vi "sort_according_to_x.vi"(8 "error in (no error)":errorcluster, 10 "points in":refnum<class "SpaceVector.lvclass">[](array[class])) -> (0 "error out":errorcluster, 2 "points out":refnum<class "SpaceVector.lvclass">[](array[class]))   [LabVIEW 2010, in "TrajectoryDL121017Hopping.lvclass"]
doc: "Sorts points according to their x coordinate."
uses:
  TrajectoryDL121017Hopping.lvclass
  common/classes/SpaceVector/SpaceVector/SpaceVector.lvclass
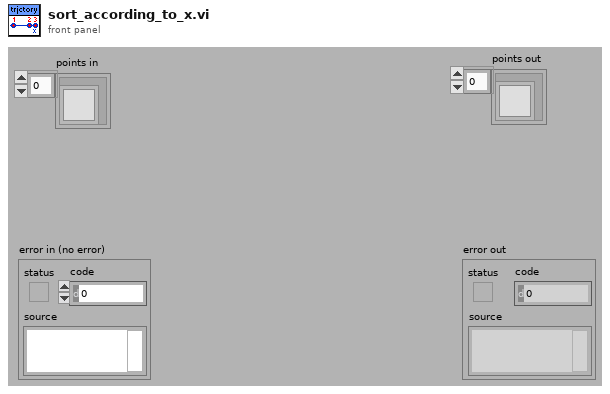
[diagram p1: front panel]
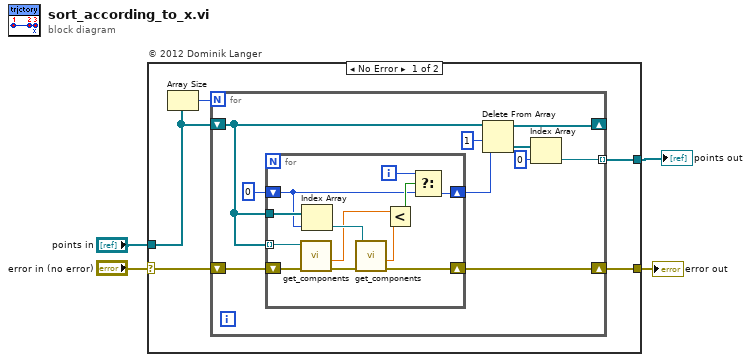
[diagram p0: block diagram]
diagram:
  n1 = case "© 2012 Dominik Langer" shown="No Error" "error in (no error)" {
    selector: "error in (no error)" -> [w9 w32]
    tunnel: [w8 w32] -> w3
    tunnel: "points in" -> [w5 _]
    tunnel: [w7 _] -> w1
    frame No Error {
      n2 = Array Size(array=w5) -> (size(s)=w6:i32)
      n3 = for {
        N: w6 -> [_]
        shift-right: [w18] -> w8
        shift-left: w9 -> [w19]
        shift-right: [w13] -> _
        shift-left: w5 -> [w16]
        tunnel: [w10] -> w7 mode=indexing
        n4 = for {
          tunnel: w16 -> [w30]
          shift-right: [w31] -> w18
          shift-left: w19 -> [w27]
          shift-right: [w20] -> w14
          shift-left: 0 -> [w21]
          tunnel: w16 -> [w28] mode=indexing
          i -> [w22]
          n5 = call "get_components.vi"("error in (no error)"=w27, "SpaceVector in"=w28) -> ("error out"=w26:errorcluster, "x"=w25:dbl[unit])  [unwired: 4 in, 4 out]
          n6 = Index Array(array=w30, index=w21) -> (element=w29:refnum<class "SpaceVector.lvclass">)
          n7 = call "get_components.vi"("error in (no error)"=w26, "SpaceVector in"=w29) -> ("error out"=w31:errorcluster, "x"=w24:dbl[unit])  [unwired: 4 in, 4 out]
          n8 = Less?(x=w25, y=w24) -> (x < y?=w23:bool)
          n9 = Select(t=w22, s=w23, f=w21) -> (s? t:f=w20:i32)
        }
        n10 = Delete From Array(array=w16, length=1, index=w14) -> (deleted portion=w12:refnum<class "SpaceVector.lvclass">[], array with subset deleted=w13:refnum<class "SpaceVector.lvclass">[])
        n11 = Index Array(array=w12, index=0) -> (element=w10:refnum<class "SpaceVector.lvclass">)
      }
    }
    frame Error {
    }
  }
  "error out" <- w3
  "points out" <- w1
